vi "main.vi"() -> ()   [LabVIEW 2021]
uses:
  NI DMM4072/NI DMM4072.lvclass
  Sim DMM/Sim DMM.lvclass
  Keysight 6700C/Keysight 6700C.lvclass
  Voltage Input/Analog Input.lvclass
  Chroma190020 HiPOT/Chroma190020 HiPOT.lvclass
  Hioki BT4560B/Hioki BT4560B.lvclass
  DMM/MultiFunction IO.lvclass
panel:
  out "Measurements":dbl[](array[numeric])
  in  "Instrument Ref 2":string
  in  "Instrument Ref":string
  out "Measurement":dbl format="%.5f"
  in  "Select":bool
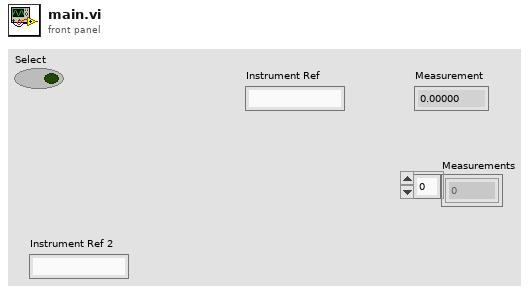
[diagram p1: front panel]
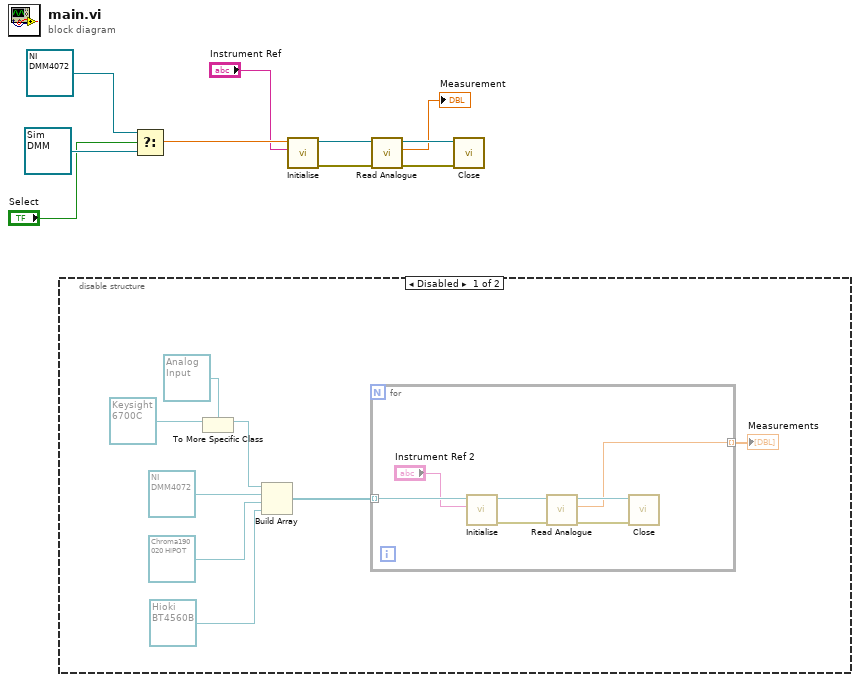
[diagram p0: block diagram]
diagram:
  n1 = disable-structure shown="Disabled" {
    frame Disabled {
      n2 = To More Specific Class(target class=refnum<class "Analog Input.lvclass"> refnum ("Analog Input.lvclass"), reference=refnum<class "Keysight 6700C.lvclass"> refnum ("Keysight 6700C.lvclass")) -> (specific class reference=w14:refnum<class "Analog Input.lvclass">)  [unwired: 1 in, 1 out]
      n3 = Build Array(w14, refnum<class "NI DMM4072.lvclass"> refnum ("NI DMM4072.lvclass"), refnum<class "Chroma190020 HiPOT.lvclass"> refnum ("Chroma190020 HiPOT.lvclass"), refnum<class "Hioki BT4560B.lvclass"> refnum ("Hioki BT4560B.lvclass")) -> (w18:refnum<class>[])
      n4 = for {
        tunnel: w18 -> [w21] mode=indexing
        tunnel: [w19] -> w11 mode=indexing
        n5 = call-dynamic "Initialise.vi"("Instrument Ref"="Instrument Ref 2", "DAQ in"=w21) -> ("error out"=w23:errorcluster, "DAQ out"=w25:refnum<class "Analog Input.lvclass">)  [unwired: 8 in]
        n6 = call-dynamic "Read Analogue.vi"("error in (no error)"=w23, "Voltage Input in"=w25) -> ("error out"=w22:errorcluster, "Measurement"=w19:dbl, "Voltage Input out"=w24:refnum<class "Analog Input.lvclass">)  [unwired: 7 in]
        n7 = call-dynamic "Close.vi"("error in (no error)"=w22, "DAQ in"=w24) -> ()  [unwired: 8 in, 2 out]
      }
      "Measurements" <- w11
    }
    frame Enabled {
    }
  }
  n8 = Select(t=refnum<class "NI DMM4072.lvclass"> refnum ("NI DMM4072.lvclass"), s="Select", f=refnum<class "Sim DMM.lvclass"> refnum ("Sim DMM.lvclass")) -> (s? t:f=w9:dbl)
  n9 = call-dynamic "Initialise.vi"("Instrument Ref"="Instrument Ref", "Instrument in"=w9) -> ("error out"=w1:errorcluster, "Instrument out"=w2:refnum<class "MultiFunction IO.lvclass">)  [unwired: 8 in]
  n10 = call-dynamic "Read Analogue.vi"("error in (no error)"=w1, "DMM in"=w2) -> ("error out"=w6:errorcluster, "Measurement"=→"Measurement":dbl, "DMM out"=w7:refnum<class "MultiFunction IO.lvclass">)  [unwired: 7 in]
  n11 = call-dynamic "Close.vi"("error in (no error)"=w6, "Instrument in"=w7) -> ()  [unwired: 8 in, 2 out]
